vi "TDT-Parse Channels and Codes.vi"(11 "Impale channel":i32[](array[numeric])) -> (0 "Labels":string[](array[string]), 2 "Sort Codes":dbl[](array[numeric]), 3 "Channels":dbl[](array[numeric]))   [LabVIEW 2015]
doc: "Converts TDT channel number and sort code pairs into a single Impale channel ID. Incorporating a sort code into Impale will break too many things, so we must send it scalar IDs. The unsorted spikes come in with a sort code of 31; we coerce that to MaxClusters + 1. MaxClusters defaults to the TDT-specified value of 5."
panel:
  in  "Max Clusters":i32=5
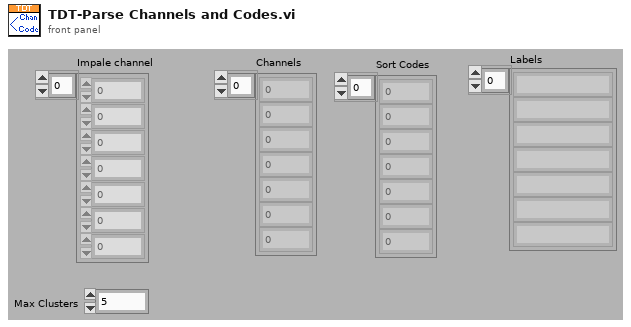
[diagram p1: front panel]
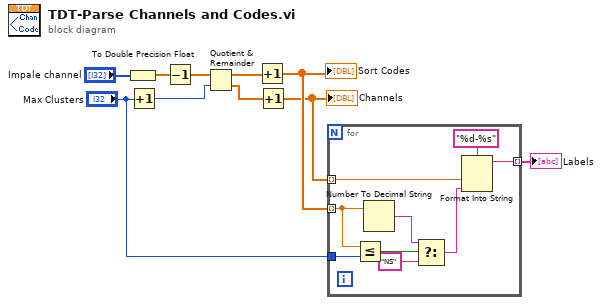
[diagram p0: block diagram]
diagram:
  n1 = To Double Precision Float(number="Impale channel") -> (double precision float=w9:dbl[])
  n2 = Increment(x="Max Clusters") -> (x+1=w7:i32)
  n3 = Decrement(x=w9) -> (x-1=w8:dbl[])
  n4 = Quotient & Remainder(x=w8, y=w7) -> (x-y*floor(x/y)=w6:dbl[], floor(x/y)=w5:dbl[])
  n5 = Increment(x=w6) -> (x+1=w4:dbl[])
  "Sort Codes" <- w4
  n6 = Increment(x=w5) -> (x+1=w3:dbl[])
  "Channels" <- w3
  n7 = for {
    tunnel: w4 -> [w14] mode=indexing
    tunnel: w3 -> [w18] mode=indexing
    tunnel: [w17] -> w1 mode=indexing
    tunnel: "Max Clusters" -> [w16]
    n8 = Less Or Equal?(x=w14, y=w16) -> (x <= y?=w15:bool)
    n9 = Number To Decimal String(number=w14) -> (decimal integer string=w13:string)  [unwired: 1 in]
    n10 = Select(t=w13, s=w15, f="NS") -> (s? t:f=w11:string)
    n11 = Format Into String(format string="%d-%s", w18, w11) -> (resulting string=w17:string)  [unwired: 2 in, 1 out]
  }
  "Labels" <- w1
